vi "Load Config_File Name Edit.vi"(8 "error in (no error)":errorcluster, 11 "Refnum in":T2) -> (0 "error out":errorcluster, 2 "File Name Edit":T1, 3 "Refnum out":T2)   [LabVIEW 2019]
uses:
  <vilib>/Utility/config.llb/Config Data RefNum.ctl
  Ctl/Ctl_Config_File Name Edit.ctl
  <vilib>/Utility/config.llb/NI_LVConfig.lvlib
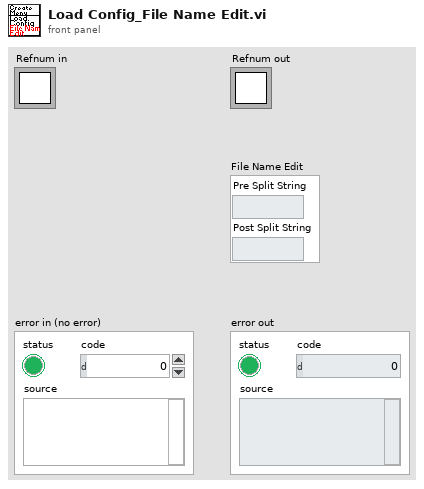
[diagram p1: front panel]
types:
  T1 = typedef "Ctl_Config_File Name Edit.ctl" = cluster{"Pre Split String":string, "Post Split String":string}
  T2 = typedef "NI_LVConfig.lvlib/Config Data RefNum.ctl" = refnum<k1>
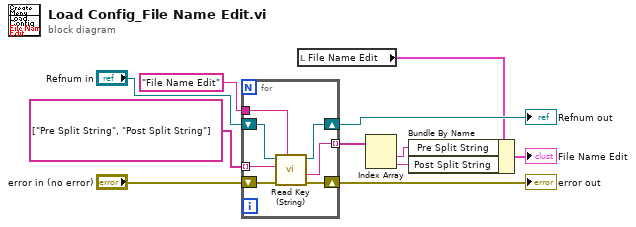
[diagram p0: block diagram]
diagram:
  n1 = for {
    tunnel: "File Name Edit" ("section") -> [w16]
    shift-right: [w15] -> w7
    shift-left: "Refnum in" -> [w17]
    shift-right: [w14] -> w6
    shift-left: "error in (no error)" -> [w18]
    tunnel: string[] ["Pre Split String", "Post Split String"] ("key") -> [w13] mode=indexing
    tunnel: [w12] -> w5 mode=indexing
    n2 = call <vilib>:"Read Key (String).vi"("section"=w16, "error in (no error)"=w18, "key"=w13, "refnum"=w17) -> ("error out"=w14:errorcluster, "value"=w12:string, "refnum out"=w15:T2)  [unwired: 4 in, 1 out]
  }
  "error out" <- w6
  "Refnum out" <- w7
  n3 = local read "File Name Edit"() -> (w1:T1)
  n4 = Index Array(array=w5) -> (element #1=w3:string, element #2=w4:string)  [unwired: 2 in]
  n5 = Bundle By Name(cluster=w1, "Pre Split String"=w3, "Post Split String"=w4) -> (→"File Name Edit":T1)
